vi "connect.vi"(8 "error in (no error)":errorcluster, 10 "VISA resource name":refnum<visa-resource-name>, 11 "keysight in":refnum<class "keysight.lvclass">) -> (0 "error out":errorcluster, 2 "VISA resource name out":refnum<visa-resource-name>, 3 "keysight out":refnum<class "keysight.lvclass">)   [LabVIEW 2015, in "keysight.lvclass"]
uses:
  keysight.lvclass
  E5071C/Agilent ENA Series/Agilent ENA Series.lvlib
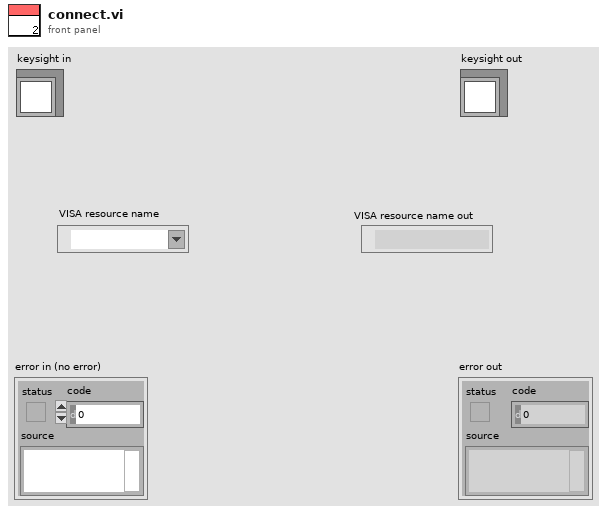
[diagram p1: front panel]
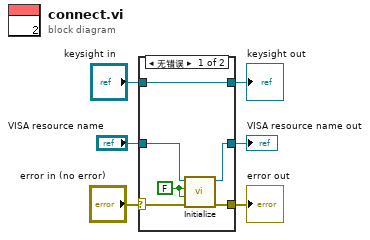
[diagram p0: block diagram]
diagram:
  n1 = case shown="无错误" "error in (no error)" {
    selector: "error in (no error)" -> [w9 w14]
    tunnel: [w11 _] -> w6
    tunnel: [w10 w14] -> w5
    tunnel: "keysight in" -> [w8 w13]
    tunnel: [w8 w13] -> w2
    tunnel: "VISA resource name" -> [w7 _]
    frame No Error {
      w12 = FALSE ("ID Query? (T: Yes)")
      n2 = call "Initialize.vi"("error in (no error)"=w9, "Reset? (T: Yes)"=w12, "ID Query? (T: Yes)"=w12, "VISA resource name"=w7) -> ("error out"=w10:errorcluster, "VISA resource name out"=w11:refnum<visa-resource-name>)  [unwired: 6 in]
    }
    frame Error {
    }
  }
  "error out" <- w5
  "keysight out" <- w2
  "VISA resource name out" <- w6
